vi "FlexRIO6581.vi"() -> ()   [LabVIEW 2013]
uses:
  Control 1.ctl
  ctl.ctl
  <vilib>/Platform/TimedLoop/XDataNode/timing_clust.ctl
  <vilib>/Platform/TimedLoop/XDataNode/nitl_modes.ctl
  <vilib>/Platform/TimedLoop/XDataNode/wakeup.ctl
  Libraries/StateControl.ctl
  Libraries/FlexRIO-Module/FlexRIO-6581/N Channels.ctl
  <vilib>/rvi/eio/common/nirviEmuTemplateMethod_errors.vi
  <vilib>/rvi/Emulation/niFpgaSctlEmulationGetInTimedLoop.vi
  <vilib>/rvi/Emulation/niFpgaEmulationReportErrorSimple.vi
  <vilib>/rvi/Emulation/niFpgaGetClockAttributes.vi
  <vilib>/rvi/Emulation/niFpgaCriticalErrorInLSC.vi
  <vilib>/rvi/FIFO/Fifo_Resource/nirvififoEmulationClearFpgaImpl.vi
  <vilib>/rvi/DataTransferAndStorage/Container/Common/niFpgaContainerGetUniqueNameForEmu.vi
  Libraries/GlobalReg.vi
  <vilib>/rvi/DataTransferAndStorage/Container/Common/niFpgaContainerExecOnDevCompGetState.vi
  <vilib>/rvi/FIFO/Fifo_Resource/nirvififoEmulationGetNumberOfElementsToReadFpgaImpl.vi
  <vilib>/rvi/interface/RandomDataEmulation/nirviRandomDataFPGAFIFO.vi
  <vilib>/rvi/interface/RandomDataEmulation/niFpgaRandomDataHandleErrors.vi
  <vilib>/rvi/eio/common/nirviEmuReportErrorAndStop.vi
  <vilib>/rvi/FIFO/Fifo_Resource/nirvififoEmulationReadFpgaImpl.vi
  <vilib>/rvi/FIFO/Fifo_Resource/nirvififoEmulationWriteFpgaImpl.vi
  <vilib>/rvi/Emulation/niFpgaProcessEmulError.vi
  <vilib>/Platform/TimedLoop/XDataNode/XDataNode.xnode
  <vilib>/eio/EIONode/EIONode.xnode
  <vilib>/rvi/DataTransferAndStorage/Container/XNode/niFpgaContainer.xnode
  <vilib>/rvi/FIFO/Fifo_Resource/nirvififoEmulationClear.vi
  <vilib>/rvi/FIFO/Fifo_Resource/niFpgaFifoEmulationRefIn.vi
  <vilib>/rvi/interface/RandomDataEmulation/nirviRandomDataFpgaReadWriteTemplate.vi
  <vilib>/Platform/TimedLoop/XDataNode/XDNodeRunTimeDep.lvlib
panel:
  in  "Cluster in":T1
  in  "Tab Control":T2(tab)=enum."Optional Resources"
  out "Platform":enum8{"FlexRIO", "cRIO", "RSeries"}(ring)
  out "FPGAVIversion":u8[](array[numeric])=[1, 1]
  out "InitDone":bool
  out "RIOAdapterCorrect":bool
  out "Fref":u32=100000000
  out "DevQualityStatus":u8
  out "DevTemp":i16=-10244
  out "DevProfile":u8 format="%x"
  in  "DAQStartStop":bool
  in  "DebugMode":bool
  out "Expected IO Module ID":u32 format="%x"
  out "InsertedIOModule ID":u32
  out "DMATtoHOSTNCh":T3[](array[typedef])=[4]
  out "DMATtoHOSTFrameType":u8[](array[numeric])
  out "DMATtoHOSTSampleSize":u8[](array[numeric])=[2]
  out "DMATtoHOSTBlockNWords":u16[](array[numeric])=[4096]
  in  "DMATtoHOSTSamplingRate0":u16=10000
  in  "DMATtoHOSTEnable0":bool
  out "DMATtoHOSTOverflows":u16
  out "auxAI5":i32
  out "auxAI4":i32
  out "auxAI3":i32
  out "auxAI2":i32
  out "auxAI1":i32
  out "auxAI0":i32
  in  "auxAO5":i32
  in  "auxAO4":i32
  in  "auxAO3":i32
  in  "auxAO2":i32
  in  "auxAO1":i32
  in  "auxAO0":i32
  out "auxDI5":bool
  out "auxDI4":bool
  out "auxDI3":bool
  out "auxDI2":bool
  out "auxDI1":bool
  out "auxDI0":bool
  in  "auxDO3":bool
  in  "auxDO4":bool
  in  "auxDO5":bool
  in  "auxDO2":bool
  in  "auxDO1":bool
  in  "auxDO0":bool
  in  "SGUpdateRate0":u32=40
  in  "SGPhase0":u32
  in  "SGFreq0":u32=100000
  in  "SGAmp0":u16
  in  "AO0":i32
  out "auxAI9":i32
  out "SGNo":u8=2 format="%x"
  out "auxAI10":i32
  in  "SGSignalType1":u8
  in  "SGAmp1":u16
  in  "SGPhase1":u32
  in  "SGFreq1":u32=100000
  in  "SGUpdateRate1":u32=40
  in  "AO1":i32
  in  "AOEnable1":bool
  out "SGFref0":u32=100000000
  out "SGFref1":u32=100000000
  in  "AOEnable0":bool
  in  "SGSignalType0":u8
  in  "auxDO6":bool
  out "DI7":bool
  out "DI6":bool
  out "DI5":bool
  out "DI4":bool
  out "DI3":bool
  out "DI2":bool
  out "DI1":bool
  out "DI0":bool
  in  "DO0":bool
  in  "DO1":bool
  in  "DO2":bool
  in  "DO3":bool
  in  "DO4":bool
  in  "DO5":bool
  in  "DO6":bool
  in  "DO7":bool
  out "toDigPort":u8
  # "Inputs"
  # "Aux \nDigital Inputs"
  # "Aux \nAnalog Inputs"
  # "Digital Inputs"
  # "Outputs"
  # "Number of WF gen"
  # "Analog Outputs"
  # "Aux Digital \nOutput"
  # "Aux Analog \nOutput"
  # "Digital Outputs"
  # "Signal Generator 1"
  # "Signal Generator 0"
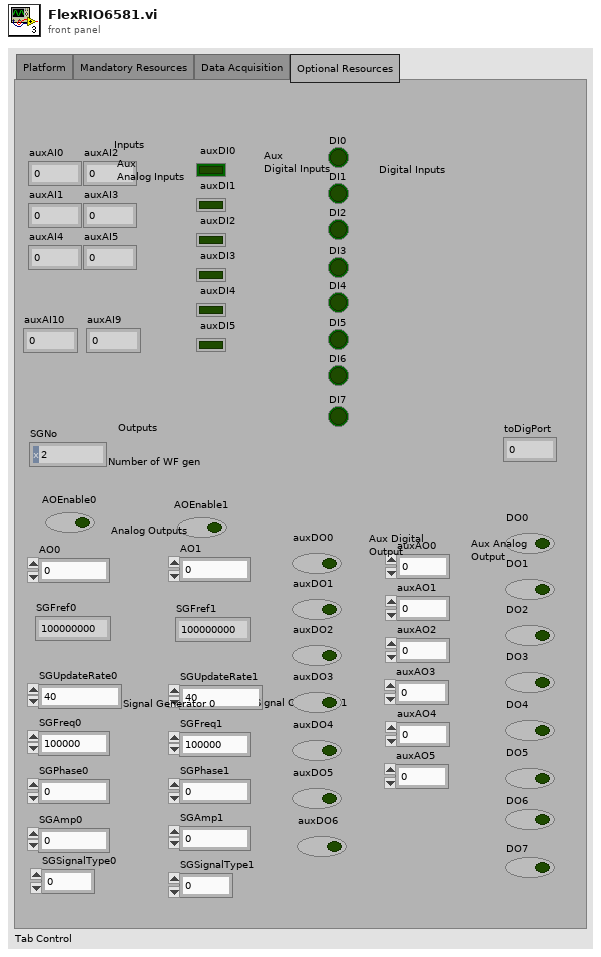
[diagram p1: front panel]
types:
  T1 = typedef "ctl.ctl" = cluster{"Number of sample in a block (0-4095)":u16, "SamplingRateN (Default 5000) (Decimation factor from ref clock)":u16, "Channels shif register up to 4 (A) ":u64, "Channels shif register up to 4 (B) ":u64, "Channels shif register up to 4 (C) ":u64, "Info shift register":u64, "ramp counter":i16, "GroupEnableN":bool, "Debug activation":bool, "Sample counter ":u64, "Decimation counter":u16, "Blocks counter":u16}
  T2 = enum32{"Platform", "Mandatory Resources", "Data Acquisition", "Optional Resources"}
  T3 = typedef "Control 1.ctl" = u16
  T4 = typedef "XDNodeRunTimeDep.lvlib/timing_clust.ctl" = cluster{"Expected End [f-1]":u64, "Actual End [f-1]":u64, "Finished Late? [f-1]":bool, "Expected End [i-1]":u64, "Actual End [i-1]":u64, "Finished Late? [i-1]":bool, "Expected Start [i]":u64, "Actual Start [i]":u64, "Expected Start [f]":u64, "Actual Start [f]":u64, "Source Name":string, "Structure Name":string, "Period":i64, "Deadline":i64, "Offset":i64, "Start":i64, "Priority":i32, "Timeout":i32, "Mode":T5, "Wakeup Reason":T6, "Error":errorcluster, "Source Type":string, "Secondary Source Type":string, "Global End Time":u64, "Global Start Time":u64, "Frame Duration":u64, "Iteration Duration":u64, "Assigned CPU":i32, "I/O Scan Engine Mode":u32}
  T5 = typedef "XDNodeRunTimeDep.lvlib/nitl_modes.ctl" = enum32{"No Change", "Process missed periods, maintain original phase", "Discard missed periods, maintain original phase", "Process missed periods, ignore original phase", "Discard missed periods, ignore original phase"}
  T6 = typedef "XDNodeRunTimeDep.lvlib/wakeup.ctl" = enum32{"Normal", "Aborted", "Asynchronous wakeup", "Timing source error", "Timed loop error", "Timeout"}
  T7 = typedef "StateControl.ctl" = enum16{"Idle", "Acq"}
  T8 = typedef "N Channels.ctl" = enum16{"0 Channels", "1 Channels", "2 Channels", "3 Channels", "4 Channels", "5 Channels", "6 Channels", "7 Channels", "8 Channels", "9 Channels", "10 Channels", "11 Channels", "12 Channels"}
  T9 = cluster{u16, u16, u64, u64, u64, u64, i16, bool, bool, u64, u16, u16}
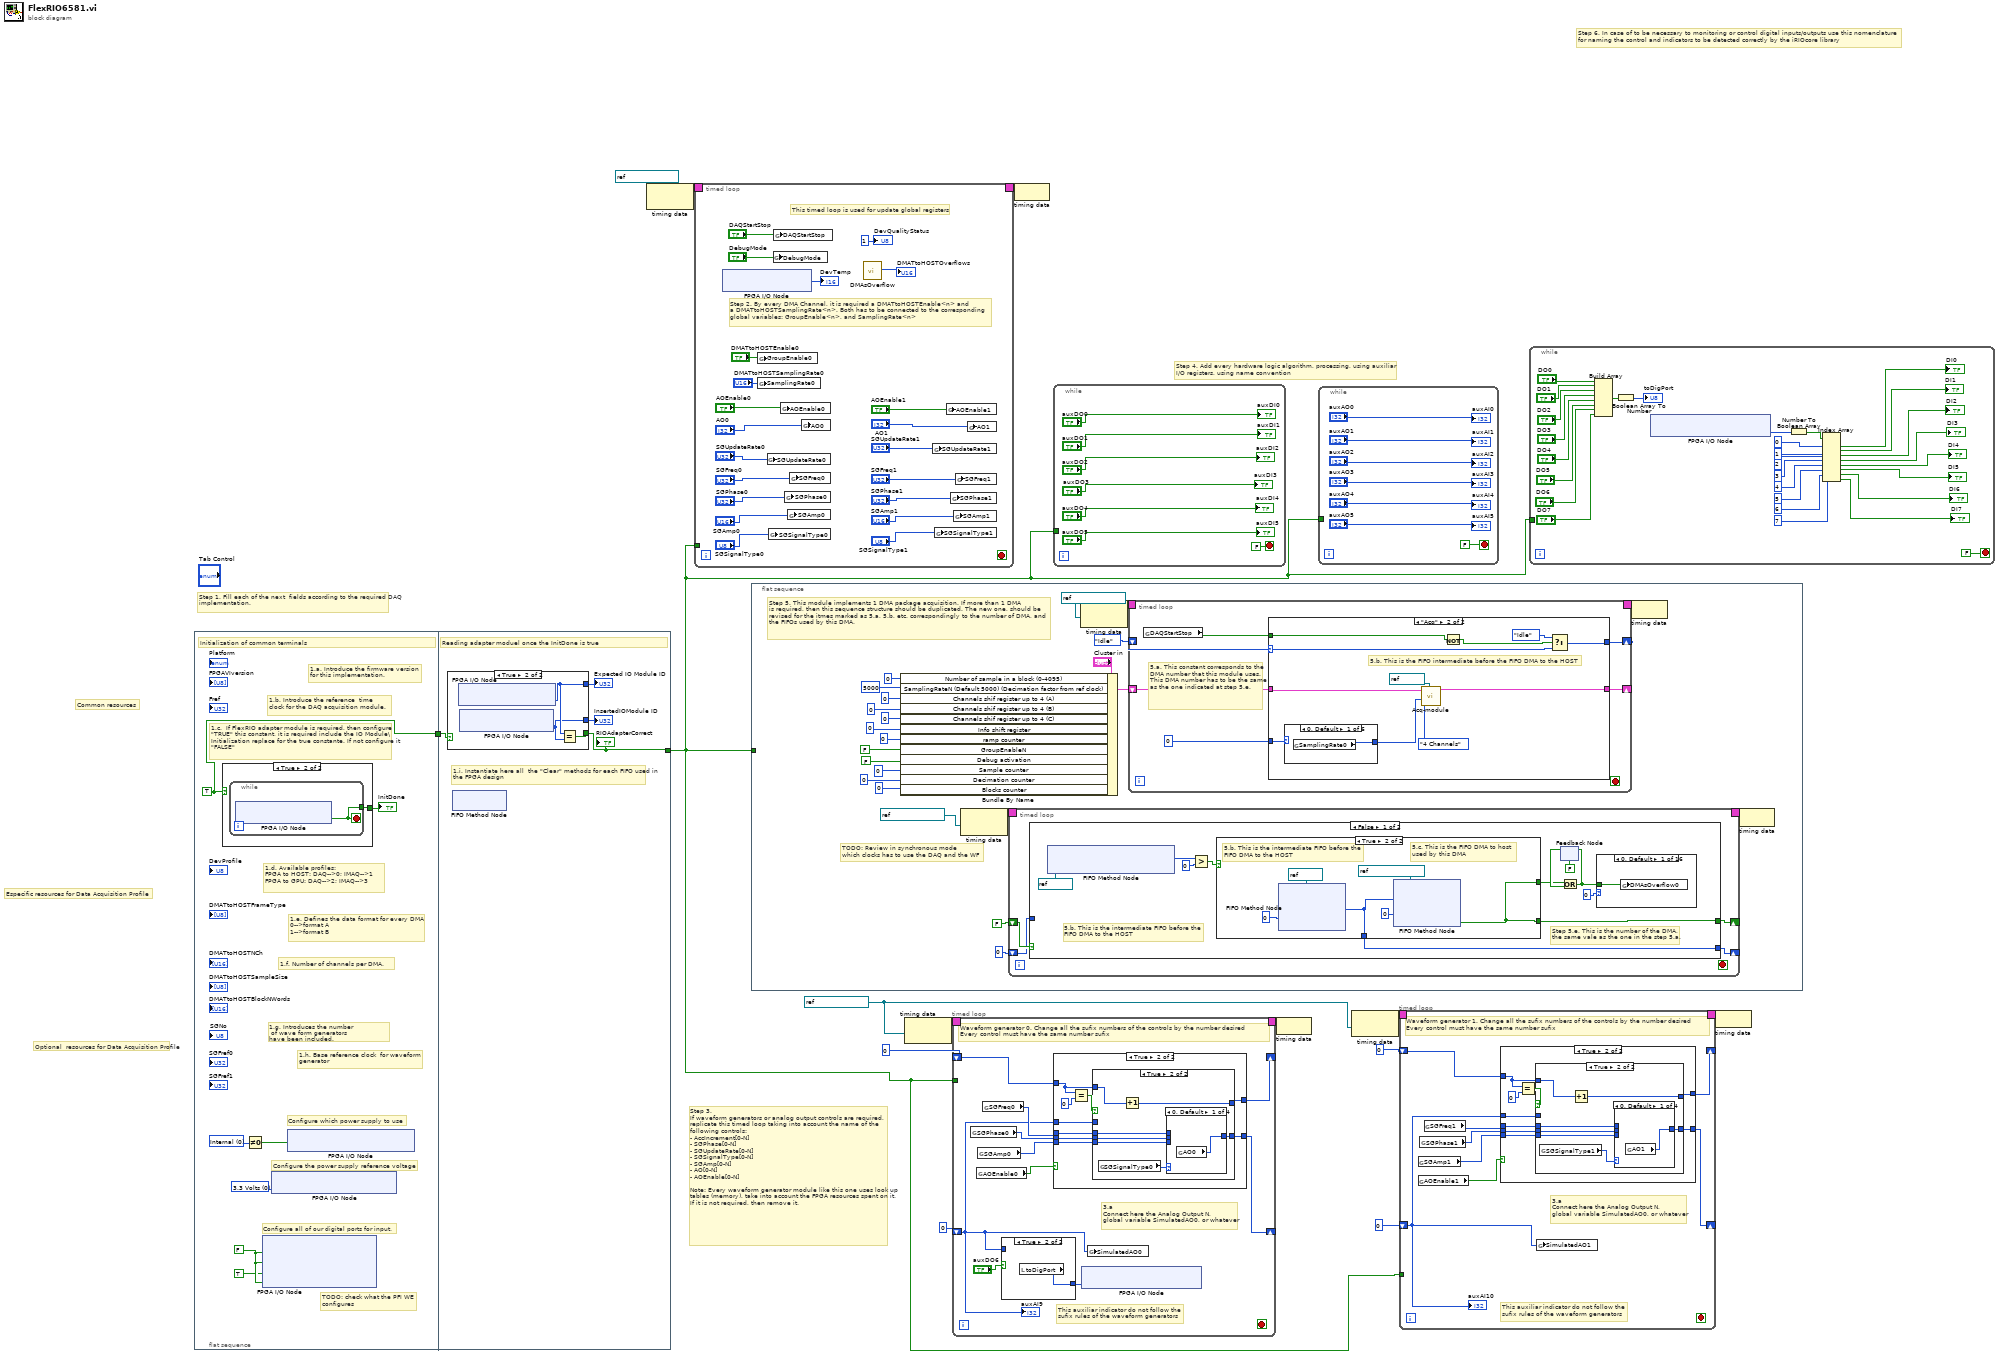
[diagram p0: block diagram]
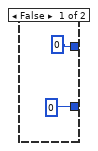
[diagram p2: hidden frame]
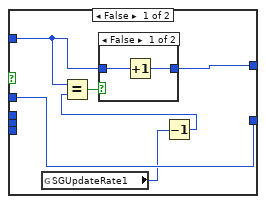
[diagram p3: hidden frame]
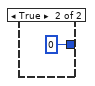
[diagram p4: hidden frame]
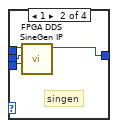
[diagram p5: hidden frame]
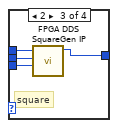
[diagram p6: hidden frame]
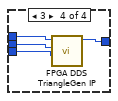
[diagram p7: hidden frame]
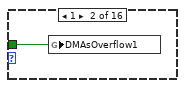
[diagram p8: hidden frame]
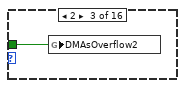
[diagram p9: hidden frame]
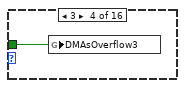
[diagram p10: hidden frame]
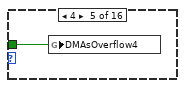
[diagram p11: hidden frame]
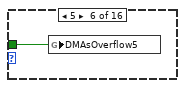
[diagram p12: hidden frame]
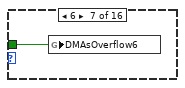
[diagram p13: hidden frame]
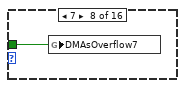
[diagram p14: hidden frame]
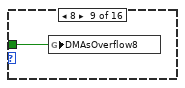
[diagram p15: hidden frame]
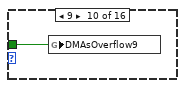
[diagram p16: hidden frame]
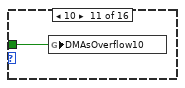
[diagram p17: hidden frame]
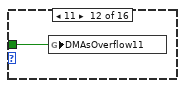
[diagram p18: hidden frame]
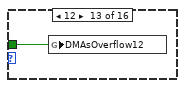
[diagram p19: hidden frame]
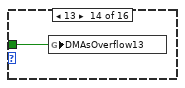
[diagram p20: hidden frame]
diagram:
  w2 = refnum<k21> "100 MHz Clock" ("Source Name")
  # "Step 3.\nIf waveform generators or analog output controls are required,\nreplicate this timed loop taking into account the name of the \nfollowing controls:\n- AccIncrement[0-N]\n- SGPhase[0-N]\n- SGUpdateRate[0-N]\n- SGSignalType[0-N]\n- SGAmp[0-N]\n- AO[0-N]\n- AOEnable[0-N]\n\nNote: Every waveform generator module like this one uses look up tables (memory), take into account the FPGA resources spent on it.  If it is not required, then remove it."
  # "Step 6. In case of to be necessary to monitoring or control digital inputs/outputs use this nomenclature\nfor naming the control and indicators to be detected correctly by the iRIOcore library"
  # "Optional  resources for Data Acquisition Profile"
  # "Especific resources for Data Acquisition Profile"
  # "Common resources"
  # "Step 4. Add every hardware logic algorithm, processing, using auxiliar \nI/O registers, using name convention"
  # "Step 1. Fill each of the next  fields according to the required DAQ implementation."
  n1 = flat-sequence {
    tunnel: [w20] -> w14
    tunnel: [w26] -> w1
    tunnel: w14 -> [w25]
    frame #0 {
      w16 = FALSE ("Terminal Block\\Port0_Write_Enable")
      w17 = u8 0 items=["3.3 Volts", "2.5 Volts", "1.8 Volts"] ("Internal Power Supply Voltage")
      w18 = u8 0 items=["Internal", "External"] ("Power Supply (Connector A)")
      w20 = TRUE
      # "TODO: check what the PFI WE\nconfigures"
      # "Configure all of our digital ports for input."
      # "Configure the power supply reference voltage"
      # "Configure which power supply to use"
      # "1.h. Base reference clock  for waveform\ngenerator"
      # "1.e. Defines the data format for every DMA\n0-->format A\n1-->format B"
      # "1.c.  If FlexRIO adapter module is required, then configure \"TRUE\" this constant, it is required include the IO Module\\Initialization replace for the true constante. If not configure it \"FALSE\""
      # "1.a. Introduce the firmware version \nfor this implementation."
      # "1.b. Introduce the reference  time \nclock for the DAQ acquisition module."
      # "1.g. Introduces the number \n of wave form generators \nhave been included."
      # "1.f. Number of channels per DMA."
      # "1.d. Available profiles: \nFPGA to HOST: DAQ-->0; IMAQ-->1\nFPGA to GPU: DAQ-->2; IMAQ-->3"
      # "Initialization of common terminals"
      n2 = case shown="True" w20 {
        tunnel: [TRUE w23] -> w21
        frame False {
        }
        frame True {
          n3 = while {
            tunnel: [w24] -> w23
            stop <- w24 stop-if-true
            n4 = xnode "FPGA I/O Node"() -> ("IO Module IO Enabled"=w24:bool)  [unwired: 1 in, 1 out]
          }
        }
      }
      "InitDone" <- w21
      n5 = Not Equal To 0?(x=w18) -> (x != 0?=w19:bool)
      n6 = xnode "FPGA I/O Node"("IO Module\\DDCA_Port0_WE"=w16, "IO Module\\DDCA_Port1_WE"=w16, "IO Module\\DDCA_Port2_WE"=TRUE ("IO Module\\DDCA_Port2_WE"), "IO Module\\DDCA_PFI_WE"=w16) -> ()  [unwired: 4 in, 4 out]
      n7 = xnode "FPGA I/O Node"("IO Module\\Local_Supply_Select"=w17) -> ()  [unwired: 1 in, 1 out]
      n8 = xnode "FPGA I/O Node"("IO Module\\DDCA_Supply_Select"=w19) -> ()  [unwired: 1 in, 1 out]
    }
    frame #1 {
      # "1.i. Instantiate here all  the \"Clear\" methods for each FIFO used in the FPGA design"
      # "Reading adapter moduel once the InitDone is true"
      n9 = case shown="True" w25 {
        tunnel: [TRUE w33] -> w26
        tunnel: [w30 w32] -> w28
        tunnel: [w30 w31] -> w27
        frame False {
          w30 = u32 0
        }
        frame True {
          n10 = xnode "FPGA I/O Node"() -> ("Expected IO Module ID"=w32:u32)  [unwired: 1 in, 1 out]
          n11 = xnode "FPGA I/O Node"() -> ("Inserted IO Module ID"=w31:u32)  [unwired: 1 in, 1 out]
          n12 = Equal?(x=w32, y=w31) -> (x = y?=w33:bool)
        }
      }
      "Expected IO Module ID" <- w28
      "InsertedIOModule ID" <- w27
      "RIOAdapterCorrect" <- w26
      n13 = xnode ("FIFO Method Node")() -> ()  [unwired: 1 in, 1 out]
    }
  }
  n14 = node-c288(refnum<k21> "100 MHz Clock" ("Source Name")) -> (w9:T4)
  n15 = timed-loop {
    timing: w9 -> [_]
    timing-out: [_] -> w8
    tunnel: w1 -> [_]
    stop <- _ stop-if-true
    # "This timed loop is used for update global registers"
    # "Step 2. By every DMA Channel, it is required a DMATtoHOSTEnable<n> and\na DMATtoHOSTSamplingRate<n>. Both has to be connected to the corresponding\nglobal variables: GroupEnable<n>, and SamplingRate<n>"
    n16 = xnode "FPGA I/O Node"() -> ("Device Temperature"=→"DevTemp":i16)  [unwired: 1 in, 1 out]
    n17 = global write "GlobalReg.vi" "GroupEnable0"("DMATtoHOSTEnable0") -> ()
    n18 = global write "GlobalReg.vi" "SamplingRate0"("DMATtoHOSTSamplingRate0") -> ()
    n19 = global write "GlobalReg.vi" "SGUpdateRate0"("SGUpdateRate0") -> ()
    n20 = global write "GlobalReg.vi" "SGSignalType0"("SGSignalType0") -> ()
    n21 = global write "GlobalReg.vi" "DebugMode"("DebugMode") -> ()
    n22 = global write "GlobalReg.vi" "DAQStartStop"("DAQStartStop") -> ()
    n23 = global write "GlobalReg.vi" "AOEnable0"("AOEnable0") -> ()
    n24 = global write "GlobalReg.vi" "SGPhase0"("SGPhase0") -> ()
    n25 = global write "GlobalReg.vi" "SGAmp0"("SGAmp0") -> ()
    n26 = global write "GlobalReg.vi" "SGFreq0"("SGFreq0") -> ()
    n27 = global write "GlobalReg.vi" "AO0"("AO0") -> ()
    n28 = call "DMAsOverflow.vi"() -> ("DMAsOverFlow"=→"DMATtoHOSTOverflows":u16)  [unwired: 11 in]
    n29 = global write "GlobalReg.vi" "SGUpdateRate1"("SGUpdateRate1") -> ()
    n30 = global write "GlobalReg.vi" "SGSignalType1"("SGSignalType1") -> ()
    n31 = global write "GlobalReg.vi" "AOEnable1"("AOEnable1") -> ()
    n32 = global write "GlobalReg.vi" "SGPhase1"("SGPhase1") -> ()
    n33 = global write "GlobalReg.vi" "SGAmp1"("SGAmp1") -> ()
    n34 = global write "GlobalReg.vi" "SGFreq1"("SGFreq1") -> ()
    n35 = global write "GlobalReg.vi" "AO1"("AO1") -> ()
    "DevQualityStatus" <- u8 1 ("DevQualityStatus")
  }
  n36 = flat-sequence {
    tunnel: w1 -> [_]
    frame #0 {
      # "TODO: Review in synchronous mode \nwhich clocks has to use the DAQ and the WF"
      # "Step 5. This module implements 1 DMA package acquisition. If more than 1 DMA \nis required, then this sequence structure should be duplicated. The new one, should be \nrevised for the itmes marked as 5.a, 5.b, etc. correspondingly to the number of DMA, and \nthe FIFOs used by this DMA."
      n37 = Bundle By Name(cluster="Cluster in", "Number of sample in a block (0-4095)"=u16 0 ("sample of block out"), "SamplingRateN (Default 5000) (Decimation factor from ref clock)"=u16 5000 ("FS1"), "Channels shif register up to 4 (A)"=u64 0, "Channels shif register up to 4 (B)"=u64 0, "Channels shif register up to 4 (C)"=u64 0, "Info shift register"=u64 0 ("Element"), "ramp counter"=i16 0, "GroupEnableN"=FALSE ("DMA1activation"), "Debug activation"=FALSE, "Sample counter"=u64 0 ("contador muestra"), "Decimation counter"=u16 0, "Blocks counter"=u16 0) -> (w60:T1)
      n38 = node-c288(refnum<k21> "100 MHz Clock" ("Source Name")) -> (w77:T4)
      n39 = timed-loop {
        timing: w77 -> [_]
        timing-out: [_] -> w76
        shift-right: [w83] -> _
        shift-left: FALSE ("Timed Out?") -> [w82]
        shift-right: [w81] -> _
        shift-left: u64 0 -> [w80]
        stop <- _ stop-if-true
        n40 = case shown="False" w82 {
          tunnel: [w88 w120] -> w83
          tunnel: [w84 w119] -> w81
          tunnel: w80 -> [_ w119]
          frame False {
            # "Step 5.e. This is the number of the DMA,\nthe same vale as the one in the step 5.a."
            # "5.b. This is the intermediate FIFO before the \nFIFO DMA to the HOST"
            n41 = xnode ("FIFO Method Node")("FIFO In"=refnum<k21> "FIFO0" ("IntermediateFIFO")) -> ("Number of Elements to Read"=w91:u32)  [unwired: 1 out]
            n42 = Greater?(x=w91, y=u32 0) -> (0:w89:bool)
            n43 = case shown="True" w89 {
              tunnel: [FALSE ("Timed Out?") w116] -> w92
              tunnel: [FALSE ("Timed Out?") w116] -> w88
              tunnel: [_ w113] -> w84
              frame False {
              }
              frame True {
                # "5.c. This is the FIFO DMA to host \nused by this DMA"
                # "5.b. This is the intermediate FIFO before the \nFIFO DMA to the HOST"
                n44 = xnode ("FIFO Method Node")("Timeout"=0, "FIFO In"=refnum<k21> "FIFO0" ("IntermediateFIFO")) -> ("Element"=w113:u64)  [unwired: 2 out]
                n45 = xnode ("FIFO Method Node")("Element"=w113, "Timeout"=0, "FIFO In"=refnum<k21> "DMATtoHOST0") -> ("Timed Out?"=w116:bool)  [unwired: 1 out]
              }
            }
            n46 = feedback #1(FALSE) -> (w93:bool)
            n47 = Or(x=w92, y=w93) -> (x .or. y?=w87:bool)
            n48 = feedback-in #1(w87) -> ()
            n49 = case shown="0, Default" i16 0 ("DMA number") {
              tunnel: w87 -> [w95 w96 w97 w98 w99 w100 w101 w102 w103 w104 w105 w106 w107 w108 w109 w110]
              frame 0, Default {
                n50 = global write "GlobalReg.vi" "DMAsOverflow0"(w95) -> ()
              }
              frame 1 {
                n51 = global write "GlobalReg.vi" "DMAsOverflow1"(w96) -> ()
              }
              frame 2 {
                n52 = global write "GlobalReg.vi" "DMAsOverflow2"(w97) -> ()
              }
              frame 3 {
                n53 = global write "GlobalReg.vi" "DMAsOverflow3"(w98) -> ()
              }
              frame 4 {
                n54 = global write "GlobalReg.vi" "DMAsOverflow4"(w99) -> ()
              }
              frame 5 {
                n55 = global write "GlobalReg.vi" "DMAsOverflow5"(w100) -> ()
              }
              frame 6 {
                n56 = global write "GlobalReg.vi" "DMAsOverflow6"(w101) -> ()
              }
              frame 7 {
                n57 = global write "GlobalReg.vi" "DMAsOverflow7"(w102) -> ()
              }
              frame 8 {
                n58 = global write "GlobalReg.vi" "DMAsOverflow8"(w103) -> ()
              }
              frame 9 {
                n59 = global write "GlobalReg.vi" "DMAsOverflow9"(w104) -> ()
              }
              frame 10 {
                n60 = global write "GlobalReg.vi" "DMAsOverflow10"(w105) -> ()
              }
              frame 11 {
                n61 = global write "GlobalReg.vi" "DMAsOverflow11"(w106) -> ()
              }
              frame 12 {
                n62 = global write "GlobalReg.vi" "DMAsOverflow12"(w107) -> ()
              }
              frame 13 {
                n63 = global write "GlobalReg.vi" "DMAsOverflow13"(w108) -> ()
              }
              frame 14 {
                n64 = global write "GlobalReg.vi" "DMAsOverflow14"(w109) -> ()
              }
              frame 15 {
                n65 = global write "GlobalReg.vi" "DMAsOverflow15"(w110) -> ()
              }
            }
          }
          frame True {
            n66 = xnode ("FIFO Method Node")("Element"=w119, "Timeout"=0) -> ("Timed Out?"=w120:bool)  [unwired: 1 in, 1 out]
          }
        }
      }
      n67 = node-c288(refnum<k21> "100 MHz Clock" ("Source Name")) -> (w79:T4)
      n68 = timed-loop {
        timing: w79 -> [_]
        timing-out: [_] -> w78
        shift-right: [w132] -> _
        shift-left: StateControl."Idle" ("Enum") -> [w133]
        shift-right: [w129] -> _
        shift-left: w60 -> [w130]
        stop <- _ stop-if-true
        # "5.a. This constant corresponds to the DMA number that this module uses. This DMA number has to be the same as the one indicated at step 5.e."
        n69 = global read "GlobalReg.vi" "DAQStartStop"() -> (w131:bool)
        n70 = case shown="\"Acq\"" w133 {
          selector: w133 -> [w143 w161]
          tunnel: w131 -> [w145 w152]
          tunnel: [w142 w160] -> w132
          tunnel: w130 -> [w141 w158]
          tunnel: [w136 w157] -> w129
          tunnel: i16 0 ("DMA number") -> [w134 w154]
          frame "Idle", Default {
            w135 = i16 0
            n71 = case shown="0, Default" w134 {
              tunnel: [w146 w147 w148 w149 w150 w151] -> w137
              frame 0, Default {
                n72 = global read "GlobalReg.vi" "GroupEnable0"() -> (w146:bool)
              }
              frame 1 {
                n73 = global read "GlobalReg.vi" "GroupEnable1"() -> (w147:bool)
              }
              frame 2 {
                n74 = global read "GlobalReg.vi" "GroupEnable2"() -> (w148:bool)
              }
              frame 3 {
                n75 = global read "GlobalReg.vi" "GroupEnable3"() -> (w149:bool)
              }
              frame 4 {
                n76 = global read "GlobalReg.vi" "GroupEnable4"() -> (w150:bool)
              }
              frame 5 {
                n77 = global read "GlobalReg.vi" "GroupEnable5"() -> (w151:bool)
              }
            }
            n78 = global read "GlobalReg.vi" "DebugMode"() -> (w138:bool)
            n79 = Bundle By Name(cluster=w141, "Number of sample in a block (0-4095)"=u16 0, "ramp counter"=u64 0, "GroupEnableN"=w137, "Debug activation"=w138, "Sample counter"=w135, "Decimation counter"=w135, "Blocks counter"=w135) -> (w136:T1)
            n80 = Select(t=StateControl."Acq" ("Enum"), s=w145, f=w143) -> (s? t:f=w142:T7)
          }
          frame "Acq" {
            # "5.b. This is the FIFO intermediate before the FIFO DMA to the HOST"
            n81 = case shown="0, Default" w154 {
              tunnel: [w163 w164 w165 w166 w167 w168] -> w159
              frame 0, Default {
                n82 = global read "GlobalReg.vi" "SamplingRate0"() -> (w163:u16)
              }
              frame 1 {
                n83 = global read "GlobalReg.vi" "SamplingRate1"() -> (w164:u16)
              }
              frame 2 {
                n84 = global read "GlobalReg.vi" "SamplingRate2"() -> (w165:u16)
              }
              frame 3 {
                n85 = global read "GlobalReg.vi" "SamplingRate3"() -> (w166:u16)
              }
              frame 4 {
                n86 = global read "GlobalReg.vi" "SamplingRate4"() -> (w167:u16)
              }
              frame 5 {
                n87 = global read "GlobalReg.vi" "SamplingRate5"() -> (w168:u16)
              }
            }
            n88 = call "Acq-module.vi"("IntermediateFIFO"=refnum<k21> "FIFO0", "NumChannels"=N_Channels."4 Channels", "SamplingRate0"=w159, "Cluster in"=w158) -> ("cluster out"=w157:T9)  [unwired: 7 in]
            n89 = Not(x=w152) -> (.not. x?=w153:bool)
            n90 = Select(t=StateControl."Idle" ("Enum"), s=w153, f=w161) -> (s? t:f=w160:T7)
          }
        }
      }
      n91 = node-c288(w78) -> ()
      n92 = node-c288(w76) -> ()
    }
  }
  n93 = node-c288(w2) -> (w13:T4)
  n94 = timed-loop {
    shift-right: [w184] -> _
    shift-left: i16 0 ("Signal Value") -> [w176]
    timing: w13 -> [_]
    timing-out: [_] -> w12
    shift-right: [w182] -> _
    shift-left: u32 0 -> [w183]
    tunnel: w1 -> [_]
    stop <- _ stop-if-true
    # "This auxiliar indicator do not follow the \nsufix rules of the waveform generators"
    # "3.a\nConnect here the Analog Output N,\nglobal variable SimulatedAO0, or whatever"
    # "Waveform generator 0. Change all the sufix numbers of the controls by the number desired\nEvery control must have the same number sufix"
    n95 = global read "GlobalReg.vi" "SGPhase0"() -> (w180:u32)
    n96 = global read "GlobalReg.vi" "AOEnable0"() -> (w178:bool)
    n97 = global read "GlobalReg.vi" "SGAmp0"() -> (w179:u16)
    n98 = global read "GlobalReg.vi" "SGFreq0"() -> (w181:u32)
    n99 = case shown="True" "auxDO6" {
      tunnel: w176 -> [w185 _]
      tunnel: [w185 w186] -> w175
      frame False {
      }
      frame True {
        n100 = local read "toDigPort"() -> (w186:u8)
      }
    }
    n101 = case shown="True" w178 {
      tunnel: w181 -> [_ w197]
      tunnel: w180 -> [_ w196]
      tunnel: w179 -> [_ w195]
      tunnel: [i16 0 w194] -> w184
      tunnel: w183 -> [_ w191]
      tunnel: [u32 0 w190] -> w182
      tunnel: w176 -> [_ w189]
      frame False {
      }
      frame True {
        n102 = Equal?(x=w191, y=u32 0) -> (x = y?=w193:bool)
        n103 = case shown="True" w193 {
          tunnel: w197 -> [_ w213]
          tunnel: w196 -> [_ w212]
          tunnel: w195 -> [_ w211]
          tunnel: [w202 w210] -> w194
          tunnel: w191 -> [w201 w209]
          tunnel: [w203 w208] -> w190
          tunnel: w189 -> [w202 _]
          frame False {
            n104 = global read "GlobalReg.vi" "SGUpdateRate0"() -> (w198:u32)
            n105 = Decrement(x=w198) -> (x-1=w199:u32)
            n106 = Equal?(x=w201, y=w199) -> (x = y?=w200:bool)
            n107 = case shown="False" w200 {
              tunnel: w201 -> [w205 _]
              tunnel: [w204 u32 0] -> w203
              frame False {
                n108 = Increment(x=w205) -> (x+1=w204:u32)
              }
              frame True {
              }
            }
          }
          frame True {
            n109 = global read "GlobalReg.vi" "SGSignalType0"() -> (w207:u8)
            n110 = Increment(x=w209) -> (x+1=w208:u32)
            n111 = case shown="0, Default" w207 {
              tunnel: w213 -> [_ w218 w222 w226]
              tunnel: w212 -> [_ w217 w221 w225]
              tunnel: w211 -> [_ w216 w220 w224]
              tunnel: [w214 w215 w219 w223] -> w210
              frame 0, Default {
                n112 = global read "GlobalReg.vi" "AO0"() -> (w214:i32)
              }
              frame 1 {
                # "singen"
                n113 = call "FPGA DDS SineGen IP.vi"("Signal Amplitude (x 2^15)"=w216, "Phase Shift"=w217, "Accumulator Increment"=w218) -> ("Signal Value"=w215:i16)  [unwired: 7 in, 1 out]
              }
              frame 2 {
                # "square"
                n114 = call "FPGA DDS SquareGen IP.vi"("Signal Amplitude (x 2^15)"=w220, "Phase Shift"=w221, "Accumulator Increment"=w222) -> ("Signal Value"=w219:i16)  [unwired: 7 in, 1 out]
              }
              frame 3 {
                n115 = call "FPGA DDS TriangleGen IP.vi"("Signal Amplitude (x 2^15)"=w224, "Phase Shift"=w225, "Accumulator Increment"=w226) -> ("Signal Value"=w223:i16)  [unwired: 7 in, 1 out]
              }
            }
          }
        }
      }
    }
    n116 = xnode "FPGA I/O Node"("IO Module\\DDCA_Port2_Write"=w175) -> ()  [unwired: 1 in, 1 out]
    n117 = global write "GlobalReg.vi" "SimulatedAO0"(w176) -> ()
    "auxAI9" <- w176
  }
  n118 = node-c288(w8) -> ()
  n119 = while {
    tunnel: w1 -> [_]
    stop <- FALSE stop-if-true
    "auxDI0" <- "auxDO0"
    "auxDI1" <- "auxDO1"
    "auxDI2" <- "auxDO2"
    "auxDI3" <- "auxDO3"
    "auxDI4" <- "auxDO4"
    "auxDI5" <- "auxDO5"
  }
  n120 = node-c288(w12) -> ()
  n121 = while {
    tunnel: w1 -> [_]
    stop <- FALSE stop-if-true
    "auxAI0" <- "auxAO0"
    "auxAI1" <- "auxAO1"
    "auxAI2" <- "auxAO2"
    "auxAI3" <- "auxAO3"
    "auxAI4" <- "auxAO4"
    "auxAI5" <- "auxAO5"
  }
  n122 = node-c288(w2) -> (w6:T4)
  n123 = timed-loop {
    shift-right: [w250] -> _
    shift-left: i16 0 ("Signal Value") -> [w247]
    timing: w6 -> [_]
    timing-out: [_] -> w5
    shift-right: [w248] -> _
    shift-left: u32 0 -> [w249]
    tunnel: w1 -> [_]
    stop <- _ stop-if-true
    # "This auxiliar indicator do not follow the \nsufix rules of the waveform generators"
    # "3.a\nConnect here the Analog Output N,\nglobal variable SimulatedAO0, or whatever"
    # "Waveform generator 1. Change all the sufix numbers of the controls by the number desired\nEvery control must have the same number sufix"
    n124 = global read "GlobalReg.vi" "SGAmp1"() -> (w244:u16)
    n125 = global read "GlobalReg.vi" "AOEnable1"() -> (w243:bool)
    n126 = global read "GlobalReg.vi" "SGPhase1"() -> (w245:u32)
    n127 = global read "GlobalReg.vi" "SGFreq1"() -> (w246:u32)
    n128 = case shown="True" w243 {
      tunnel: w246 -> [_ w261]
      tunnel: w245 -> [_ w260]
      tunnel: w244 -> [_ w259]
      tunnel: [i16 0 w258] -> w250
      tunnel: w249 -> [_ w255]
      tunnel: [u32 0 w254] -> w248
      tunnel: w247 -> [_ w253]
      frame False {
      }
      frame True {
        n129 = Equal?(x=w255, y=u32 0) -> (x = y?=w257:bool)
        n130 = case shown="True" w257 {
          tunnel: w261 -> [_ w277]
          tunnel: w260 -> [_ w276]
          tunnel: w259 -> [_ w275]
          tunnel: [w266 w274] -> w258
          tunnel: w255 -> [w265 w273]
          tunnel: [w267 w272] -> w254
          tunnel: w253 -> [w266 _]
          frame False {
            n131 = global read "GlobalReg.vi" "SGUpdateRate1"() -> (w262:u32)
            n132 = Decrement(x=w262) -> (x-1=w263:u32)
            n133 = Equal?(x=w265, y=w263) -> (x = y?=w264:bool)
            n134 = case shown="False" w264 {
              tunnel: w265 -> [w269 _]
              tunnel: [w268 u32 0] -> w267
              frame False {
                n135 = Increment(x=w269) -> (x+1=w268:u32)
              }
              frame True {
              }
            }
          }
          frame True {
            n136 = global read "GlobalReg.vi" "SGSignalType1"() -> (w271:u8)
            n137 = Increment(x=w273) -> (x+1=w272:u32)
            n138 = case shown="0, Default" w271 {
              tunnel: w277 -> [_ w282 w286 w290]
              tunnel: w276 -> [_ w281 w285 w289]
              tunnel: w275 -> [_ w280 w284 w288]
              tunnel: [w278 w279 w283 w287] -> w274
              frame 0, Default {
                n139 = global read "GlobalReg.vi" "AO1"() -> (w278:i32)
              }
              frame 1 {
                # "singen"
                n140 = call "FPGA DDS SineGen IP.vi"("Signal Amplitude (x 2^15)"=w280, "Phase Shift"=w281, "Accumulator Increment"=w282) -> ("Signal Value"=w279:i16)  [unwired: 7 in, 1 out]
              }
              frame 2 {
                # "square"
                n141 = call "FPGA DDS SquareGen IP.vi"("Signal Amplitude (x 2^15)"=w284, "Phase Shift"=w285, "Accumulator Increment"=w286) -> ("Signal Value"=w283:i16)  [unwired: 7 in, 1 out]
              }
              frame 3 {
                n142 = call "FPGA DDS TriangleGen IP.vi"("Signal Amplitude (x 2^15)"=w288, "Phase Shift"=w289, "Accumulator Increment"=w290) -> ("Signal Value"=w287:i16)  [unwired: 7 in, 1 out]
              }
            }
          }
        }
      }
    }
    n143 = global write "GlobalReg.vi" "SimulatedAO1"(w247) -> ()
    "auxAI10" <- w247
  }
  n144 = while {
    tunnel: w1 -> [_]
    stop <- FALSE stop-if-true
    n145 = Build Array("DO0", "DO1", "DO2", "DO3", "DO4", "DO5", "DO6", "DO7") -> (w312:bool[])
    n146 = Boolean Array To Number(Boolean array=w312) -> (number=→"toDigPort":u8)
    n147 = xnode "FPGA I/O Node"() -> ("IO Module\\DDCA_Port1_Read"=w310:u8)  [unwired: 1 in, 1 out]
    n148 = Number To Boolean Array(number=w310) -> (Boolean array=w309:bool[])
    n149 = Index Array(array=w309, index #1=0 ("index"), index #2=1 ("index"), index #3=2 ("index"), index #4=3 ("index"), index #5=4 ("index"), index #6=5 ("index"), index #7=6 ("index"), index #8=7 ("index")) -> (element #1=→"DI0":bool, element #2=→"DI1":bool, element #3=→"DI2":bool, element #4=→"DI3":bool, element #5=→"DI4":bool, element #6=→"DI5":bool, element #7=→"DI6":bool, element #8=→"DI7":bool)
  }
  n150 = node-c288(w5) -> ()
